vi "Delete Item By Index.vi"(8 "错误输入":errorcluster, 10 "Index":i32, 11 "Mlistbox Ref":refnum<vi>) -> (0 "错误输出":errorcluster, 3 "Mlistbox Ref Dup":refnum<vi>)   [LabVIEW 2012, in "Mlistbox Tools.lvlib"]
uses:
  Mlistbox Tools.lvlib
  ListBox/Custom Type/Read and Write Mode.ctl
  Property/Set and Get ItemNames.vi
  ListBox/Listbox Tool.lvlib
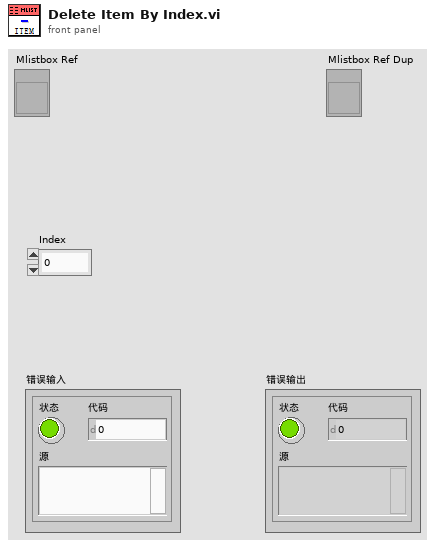
[diagram p1: front panel]
types:
  T1 = typedef "Listbox Tool.lvlib/Read and Write Mode.ctl" = enum16{"Read", "Write"}
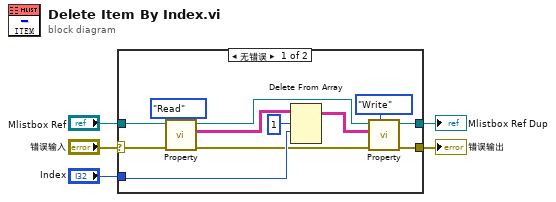
[diagram p0: block diagram]
diagram:
  n1 = case shown="无错误" "错误输入" {
    selector: "错误输入" -> [w14 w19]
    tunnel: [w12 w19] -> w4
    tunnel: "Mlistbox Ref" -> [w17 w18]
    tunnel: [w13 w18] -> w2
    tunnel: "Index" -> [w9 _]
    frame No Error {
      n2 = call-poly "Property.vi"("Mode"=Read_and_Write_Mode."Read", "错误输入"=w14, "Mlistbox Ref"=w17) -> ("错误输出"=w6:errorcluster, "ItemNames Out"=w10:string[][], "Mlistbox Ref Dup"=w11:refnum<vi>)  [unwired: 6 in]
      n3 = Delete From Array(array=w10, length=1 ("长度"), index (row)=w9) -> (array with subset deleted=w7:string[][])  [unwired: 1 in, 1 out]
      n4 = call-poly "Property.vi"("Mode"=Read_and_Write_Mode."Write", "错误输入"=w6, "ItemNames In"=w7, "Mlistbox Ref"=w11) -> ("错误输出"=w12:errorcluster, "Mlistbox Ref Dup"=w13:refnum<vi>)  [unwired: 5 in, 1 out]
    }
    frame Error {
    }
  }
  "Mlistbox Ref Dup" <- w2
  "错误输出" <- w4
